vi "niRFUtil CONV 1 Ohm Watt to 1 Ohm Voltage (real array).vi"(7 "Real Array (W)":T1 min=0 max=127 format="%.2f") -> (8 "Real Array (V)":T1 min=0 max=127 format="%.2f")   [LabVIEW 2015, in "niRFUtil.lvlib"]
doc: "(c) Copyright 2006, National Instruments, Inc. This VI may not be duplicated, sold, or distributed without written consent from National Instruments."
uses:
  niRFUtil.lvlib
  Includes/niRFUtil INC Real Array.ctl
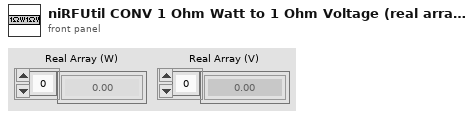
[diagram p1: front panel]
types:
  T1 = typedef "niRFUtil.lvlib/niRFUtil INC Real Array.ctl" = sgl[]
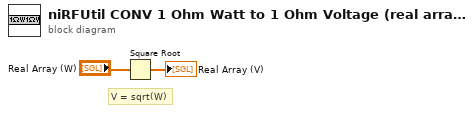
[diagram p0: block diagram]
diagram:
  # "V = sqrt(W)"
  n1 = Square Root(x="Real Array (W)") -> (sqrt(x)=→"Real Array (V)":T1)
